vi "Autonomous Independent.vi"   [LabVIEW 2018]
doc: "This VI is called when autonomous begins, and will automatically be terminated when autonomous ends. You can carry out timed or sensor driven robot movement independently without needing to return to the caller."
uses:
  <vilib>/Rock Robotics/WPI/Ultrasonic/WPI_UltrasonicRangeUnits.ctl
  <vilib>/Rock Robotics/WPI/Utilities/WPI_GetSetVariantRefNum.vi
  <vilib>/Rock Robotics/Network Tables/NT Read String.vi
  <vilib>/Rock Robotics/Network Tables/NT Write Numeric Array.vi
  <vilib>/Rock Robotics/WPI/Ultrasonic/WPI_SonarSRF04DigitalRefNum Registry Get.vi
  <vilib>/Rock Robotics/WPI/RobotDrive/WPI_RobotDriveArcadeDrive_Standard(NoSaturation).vi
  <vilib>/Rock Robotics/WPI/Ultrasonic/WPI_SonarSRF04DigitalGetRange.vi
panel:
  # "Be sure to right-click and choose Data Operations>>Make Current Value default if you want to save the array values with the VI"
types:
  T1 = typedef "WPI_JoystickDevRef.ctl" = cluster{"Device":T2}
  T2 = typedef "WPI_JoystickDeviceEnum.ctl" = enum16{"USB 0", "USB 1", "USB 2", "USB 3", "USB 4", "USB 5"}
  T3 = typedef "WPI_UltrasonicRangeUnits.ctl" = enum16{"inches", "mm"}
  T4 = typedef "WPI_UltrasonicDeviceRef.ctl" = cluster{"DevStatus":errorcluster, "Ping Channel":T5, "Echo Channel":T5, "CntIndex":T6}
  T5 = typedef "FPGA_DIOChannel.ctl" = enum8{"DIO 0", "DIO 1", "DIO 2", "DIO 3", "DIO 4", "DIO 5", "DIO 6", "DIO 7", "DIO 8", "DIO 9", "DIO MXP 0", "DIO MXP 1", "DIO MXP 2", "DIO MXP 3", "DIO MXP 4", "DIO MXP 5", "DIO MXP 6", "DIO MXP 7", "DIO MXP 8", "DIO MXP 9", "DIO MXP 10", "DIO MXP 11", "DIO MXP 12", "DIO MXP 13", "DIO MXP 14", "DIO MXP 15", "SPI Port CS1", "SPI Port CS2", "SPI Port CS3", "SPI Port MISO", "SPI Port MOSI", "Invalid"}
  T6 = typedef "FPGA_CounterCtrSystemIndex.ctl" = enum8{"Ctr 0", "Ctr 1", "Ctr 2", "Ctr 3", "Ctr 4", "Ctr 5", "Ctr 6", "Ctr 7", "Invalid"}
  T7 = typedef "WPI_ServoDeviceRef.ctl" = cluster{"DeviceStatus":errorcluster, "PWM Channel":T8, "DeadBand":T9}
  T8 = typedef "FPGA_DIOPWMChannel.ctl" = enum8{"PWM 0", "PWM 1", "PWM 2", "PWM 3", "PWM 4", "PWM 5", "PWM 6", "PWM 7", "PWM 8", "PWM 9", "PWM MXP 0", "PWM MXP 1", "PWM MXP 2", "PWM MXP 3", "PWM MXP 4", "PWM MXP 5", "PWM MXP 6", "PWM MXP 7", "PWM MXP 8", "PWM MXP 9", "Invalid"}
  T9 = typedef "WPI_PWMDeadband.ctl" = cluster{"Name":string, "maxPositivePwm":i32, "minPositivePwm":i32, "centerPwm":i32, "maxNegativePwm":i32, "minNegativePwm":i32, "angularRange":u16}
  T10 = typedef "WPI_RobotDriveDevRef.ctl" = cluster{"DevStatus":errorcluster, "Motors[]":T11[], "Square Inputs":bool, "Max Output":dbl}
  T11 = typedef "WPI_MotorControlDeviceRef.ctl" = cluster{"DeviceStatus":errorcluster, "Type":T12, "PWM":cluster{"PWM Channel":T8, "DeadBand":T9}, "CAN":cluster{"Device Number":u8, "SetOutput VI Ref":variant, "GetOutput VI Ref":variant, "Enable VI Ref":variant, "Disable VI Ref":variant, "Data":variant}, "Invert":bool, "DIO PWM":cluster{"PWM \"Enable\" Channel":T8, "DIOChannel":T5, "PWM Rate":dbl}}
  T12 = typedef "WPI_MotorControlType.ctl" = enum16{"PWM", "CAN", "DIO PWM"}
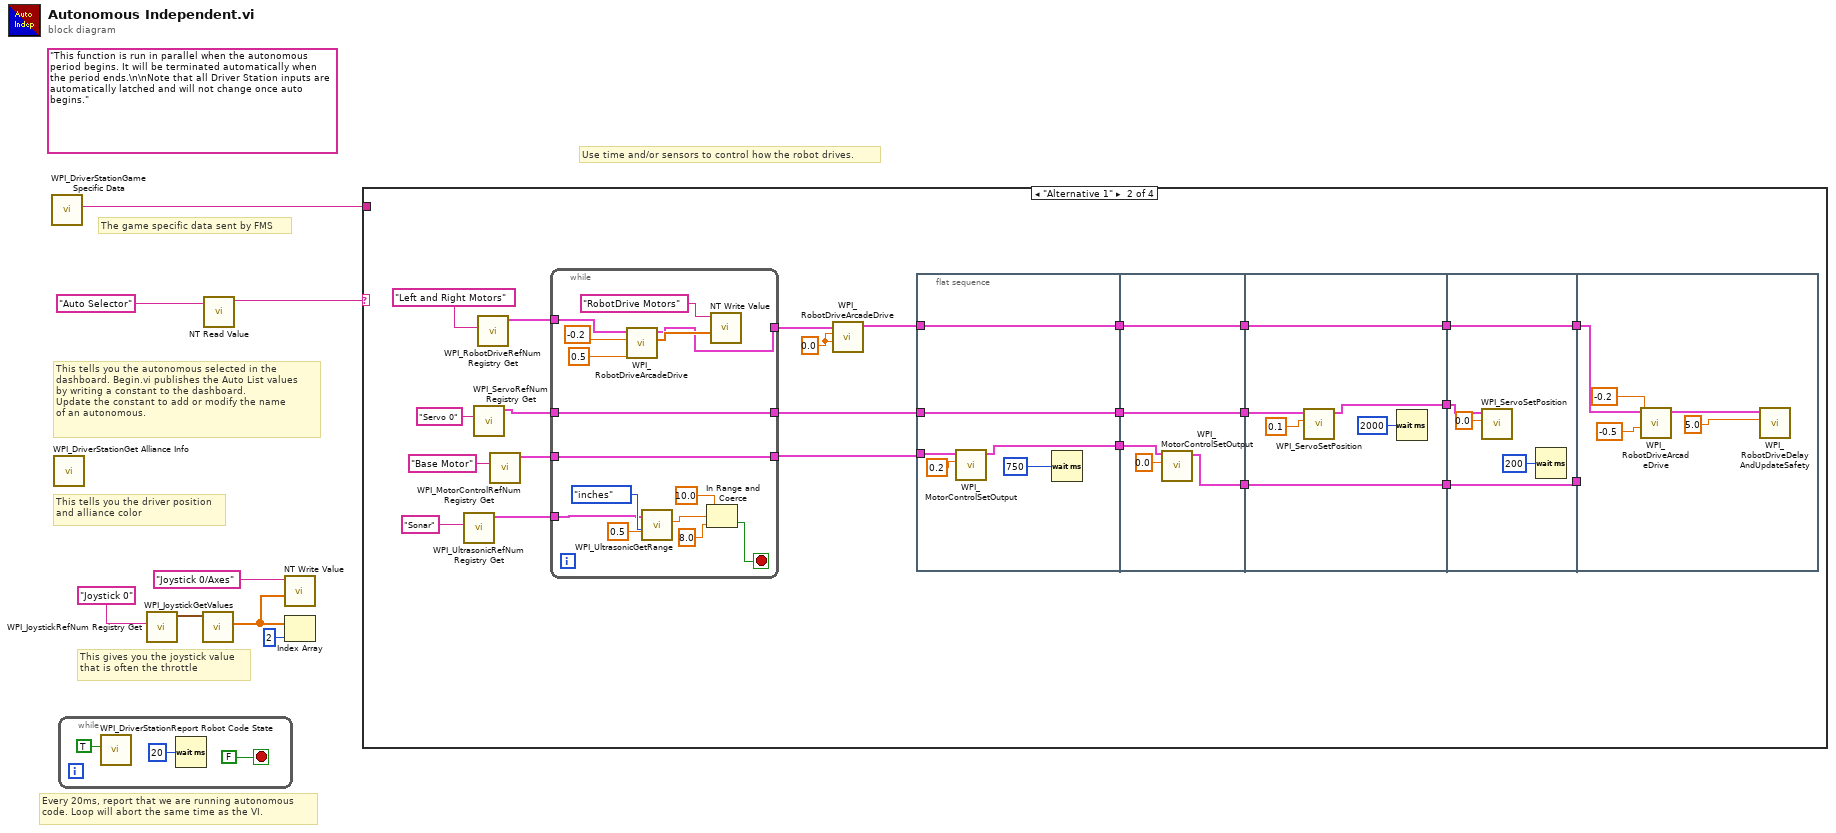
[diagram p0: block diagram]
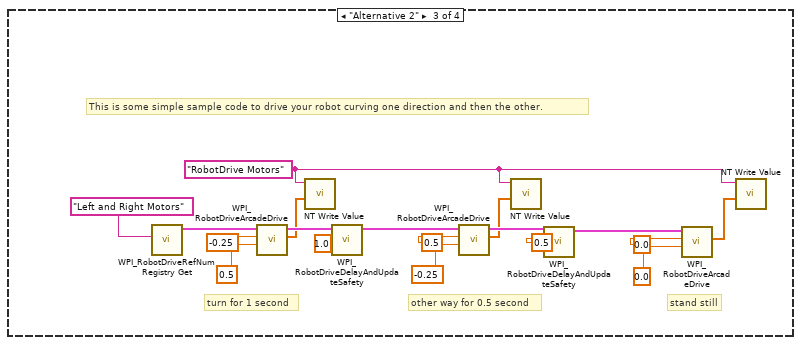
[diagram p3: hidden frame]
diagram:
  (unwired) "This function is run in parallel when the autonomous period begins. It will be terminated automatically when the period ends.\n\nNote that all Driver Station inputs are automatically latched and will not change once auto begins."
  # "The game specific data sent by FMS"
  # "This tells you the autonomous selected in the \ndashboard. Begin.vi publishes the Auto List values\nby writing a constant to the dashboard.\nUpdate the constant to add or modify the name\nof an autonomous."
  # "Every 20ms, report that we are running autonomous\ncode. Loop will abort the same time as the VI."
  # "This gives you the joystick value\nthat is often the throttle"
  # "Use time and/or sensors to control how the robot drives."
  # "This tells you the driver position\nand alliance color"
  n1 = call <vilib>:"WPI_DriverStationGame Specific Data.vi"() -> ("Game Specific Data"=w1:string)  [unwired: 11 in]
  n2 = call <vilib>:"WPI_DriverStationGet Alliance Info.vi"() -> ()  [unwired: 12 out]
  n3 = while {
    stop <- FALSE stop-if-true
    n4 = call <vilib>:"WPI_DriverStationReport Robot Code State.vi"("Autonomous"=TRUE) -> ()  [unwired: 10 in, 1 out]
    n5 = Wait (ms)(milliseconds to wait=u32 20) -> ()  [unwired: 1 out]
  }
  n6 = call <vilib>:"WPI_JoystickRefNum Registry Get.vi"("refnum name"="Joystick 0") -> ("JoystickDevRef"=w7:T1)  [unwired: 1 in, 9 out]
  n7 = call <vilib>:"WPI_JoystickGetValues.vi"("JoystickDevRef"=w7) -> ("Axes"=w3:dbl[])  [unwired: 6 in, 4 out]
  n8 = call-poly <vilib>:"NT Read Value.vi"("Name"="Auto Selector") -> ("String"=w4:string)  [unwired: 9 in, 1 out]
  n9 = call-poly <vilib>:"NT Write Value.vi"("Numeric Array"=w3, "Name"="Joystick 0/Axes") -> ()  [unwired: 9 in, 1 out]
  n10 = Index Array(array=w3, index=2) -> ()  [unwired: 1 out]
  n11 = case shown="\"Alternative 1\"" w4 {
    tunnel: w1 -> [_ _ _ _]
    frame Default {
    }
    frame "Alternative 1" {
      w30 = 0.0
      n12 = call-poly <vilib>:"WPI_UltrasonicRefNum Registry Get.vi"("refnum name"="Sonar") -> ("SonarSRF04DevRef"=w34:T4)  [unwired: 9 in, 1 out]
      n13 = call <vilib>:"WPI_ServoRefNum Registry Get.vi"("refnum name"="Servo 0") -> ("ServoDeviceRef"=w27:T7)  [unwired: 9 in, 1 out]
      n14 = call <vilib>:"WPI_RobotDriveRefNum Registry Get.vi"("refnum name"="Left and Right Motors") -> ("RobotDriveDevRef"=w32:T10)  [unwired: 1 in, 9 out]
      n15 = call <vilib>:"WPI_MotorControlRefNum Registry Get.vi"("refnum name"="Base Motor") -> ("MotorControlDevRef"=w24:T11)  [unwired: 9 in, 1 out]
      n16 = while {
        tunnel: w34 -> [w75]
        tunnel: w32 -> [w70]
        tunnel: [w65] -> w31
        tunnel: [w64] -> w28
        tunnel: w27 -> [w64]
        tunnel: [w63] -> w25
        tunnel: w24 -> [w63]
        stop <- w71 stop-if-true
        n17 = call-poly <vilib>:"WPI_RobotDriveArcadeDrive.vi"("Y axis value"=0.5, "X axis value"=-0.2, "RobotDriveDevRef"=w70) -> ("Motor Values"=w66:dbl[], "RobotDriveDevRef"=w65:T10)  [unwired: 6 in, 1 out]
        n18 = call-poly <vilib>:"WPI_UltrasonicGetRange.vi"("Range Units"=WPI_UltrasonicRangeUnits."inches", "ping time (s)"=sgl 0.5, "SonarSRF04DevRef"=w75) -> ("Distance"=w74:dbl)  [unwired: 6 in, 2 out]
        n19 = In Range and Coerce(upper limit=10.0, x=w74, lower limit=8.0) -> (In Range?=w71:bool)  [unwired: 1 out]
        n20 = call-poly <vilib>:"NT Write Value.vi"("Numeric Array"=w66, "Name"="RobotDrive Motors") -> ()  [unwired: 9 in, 1 out]
      }
      n21 = call-poly <vilib>:"WPI_RobotDriveArcadeDrive.vi"("Y axis value"=w30, "X axis value"=w30, "RobotDriveDevRef"=w31) -> ("RobotDriveDevRef"=w12:T10)  [unwired: 6 in, 2 out]
      n22 = flat-sequence {
        tunnel: w28 -> [w41]
        tunnel: [w41] -> w23
        tunnel: w25 -> [w40]
        tunnel: [w37] -> w21
        tunnel: [w36] -> w13
        tunnel: w12 -> [w36]
        tunnel: w23 -> [w46]
        tunnel: [w46] -> w22
        tunnel: w21 -> [w45]
        tunnel: [w43] -> w17
        tunnel: [w42] -> w14
        tunnel: w13 -> [w42]
        tunnel: w22 -> [w52]
        tunnel: [w49] -> w20
        tunnel: [w48] -> w18
        tunnel: w17 -> [w48]
        tunnel: [w47] -> w15
        tunnel: w14 -> [w47]
        tunnel: w20 -> [w57]
        tunnel: [w54] -> w19
        tunnel: w18 -> [w54]
        tunnel: [w53] -> w16
        tunnel: w15 -> [w53]
        tunnel: w19 -> [_]
        tunnel: w16 -> [w62]
        frame #0 {
          n23 = call <vilib>:"WPI_MotorControlSetOutput.vi"("Output"=0.2, "MotorControlDevRef"=w40) -> ("MotorControlDevRef"=w37:T11)  [unwired: 7 in, 2 out]
          n24 = Wait (ms)(milliseconds to wait=750) -> ()  [unwired: 1 out]
        }
        frame #1 {
          n25 = call <vilib>:"WPI_MotorControlSetOutput.vi"("Output"=0.0, "MotorControlDevRef"=w45) -> ("MotorControlDevRef"=w43:T11)  [unwired: 7 in, 2 out]
        }
        frame #2 {
          n26 = call <vilib>:"WPI_ServoSetPosition.vi"("Position"=0.1, "ServoDeviceRef"=w52) -> ("ServoDeviceRef"=w49:T7)  [unwired: 8 in, 1 out]
          n27 = Wait (ms)(milliseconds to wait=u32 2000) -> ()  [unwired: 1 out]
        }
        frame #3 {
          n28 = call <vilib>:"WPI_ServoSetPosition.vi"("Position"=0.0, "ServoDeviceRef"=w57) -> ()  [unwired: 8 in, 2 out]
          n29 = Wait (ms)(milliseconds to wait=u32 200) -> ()  [unwired: 1 out]
        }
        frame #4 {
          n30 = call-poly <vilib>:"WPI_RobotDriveArcadeDrive.vi"("Y axis value"=-0.5, "X axis value"=-0.2, "RobotDriveDevRef"=w62) -> ("RobotDriveDevRef"=w59:T10)  [unwired: 6 in, 2 out]
          n31 = call <vilib>:"WPI_RobotDriveDelayAndUpdateSafety.vi"("Delay (s)"=5.0, "RobotDriveDevRef"=w59) -> ()  [unwired: 8 in, 2 out]
        }
      }
    }
    frame "Alternative 2" {
      w79 = "RobotDrive Motors" ("Name")
      # "This is some simple sample code to drive your robot curving one direction and then the other."
      # "stand still"
      # "other way for 0.5 second"
      # "turn for 1 second"
      n32 = call <vilib>:"WPI_RobotDriveRefNum Registry Get.vi"("refnum name"="Left and Right Motors") -> ("RobotDriveDevRef"=w95:T10)  [unwired: 1 in, 9 out]
      n33 = call-poly <vilib>:"WPI_RobotDriveArcadeDrive.vi"("Y axis value"=0.5 ("X axis value"), "X axis value"=-0.25, "RobotDriveDevRef"=w95) -> ("Motor Values"=w78:dbl[], "RobotDriveDevRef"=w88:T10)  [unwired: 1 in, 6 out]
      n34 = call-poly <vilib>:"NT Write Value.vi"("Numeric Array"=w78, "Name"=w79) -> ()  [unwired: 9 in, 1 out]
      n35 = call <vilib>:"WPI_RobotDriveDelayAndUpdateSafety.vi"("Delay (s)"=1.0, "RobotDriveDevRef"=w88) -> ("RobotDriveDevRef 2"=w89:T10)  [unwired: 8 in, 1 out]
      n36 = call-poly <vilib>:"WPI_RobotDriveArcadeDrive.vi"("Y axis value"=-0.25 ("X axis value"), "X axis value"=0.5, "RobotDriveDevRef"=w89) -> ("Motor Values"=w80:dbl[], "RobotDriveDevRef"=w90:T10)  [unwired: 1 in, 6 out]
      n37 = call-poly <vilib>:"NT Write Value.vi"("Numeric Array"=w80, "Name"=w79) -> ()  [unwired: 9 in, 1 out]
      n38 = call <vilib>:"WPI_RobotDriveDelayAndUpdateSafety.vi"("Delay (s)"=0.5, "RobotDriveDevRef"=w90) -> ("RobotDriveDevRef 2"=w91:T10)  [unwired: 8 in, 1 out]
      n39 = call-poly <vilib>:"WPI_RobotDriveArcadeDrive.vi"("Y axis value"=0.0 ("X axis value"), "X axis value"=0.0, "RobotDriveDevRef"=w91) -> ("Motor Values"=w81:dbl[])  [unwired: 1 in, 7 out]
      n40 = call-poly <vilib>:"NT Write Value.vi"("Numeric Array"=w81, "Name"=w79) -> ()  [unwired: 9 in, 1 out]
    }
    frame "Your Turn" {
    }
  }
